vi "slider.vi"(0 "Slide":dbl(slide) scale=0.0..10.0, 6 "Playback":bool, 8 "Stop":bool, 11 "error in (no error)":errorcluster) -> (4 "Display Text":string caption="String 2", 15 "error out":errorcluster)   [LabVIEW 2023, in "Task_1.lvlib"]
doc: "Slider to set the value."
uses:
  Task_1.lvlib
  Control/Operations.ctl
  Control/Data.ctl
  Control/Control 7.ctl
  Control/State.ctl
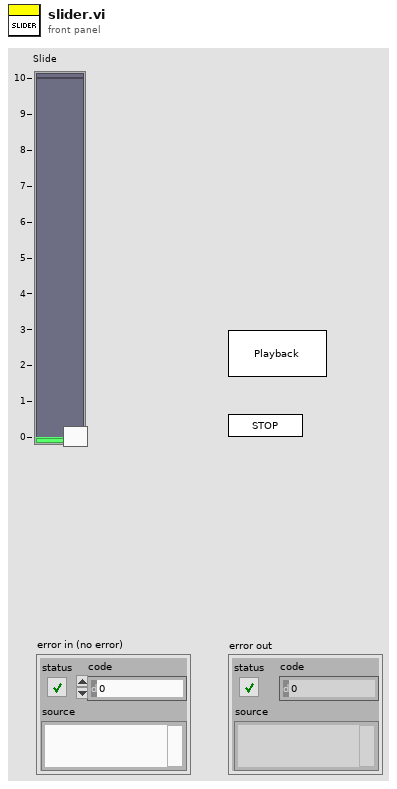
[diagram p1: front panel]
types:
  T1 = typedef "Control 7.ctl" = cluster{"State":T2, "Data":dbl[], "Index":i32}
  T2 = typedef "Task_1.lvlib/State.ctl" = enum16{"Idle", "Playback", "Record"}
  T3 = typedef "Task_1.lvlib/Data.ctl" = cluster{"Created?":bool, "Data":dbl}
  T4 = typedef "Task_1.lvlib/Operations.ctl" = enum16{"Create", "Gen_ref", "Generate", "Destroy"}
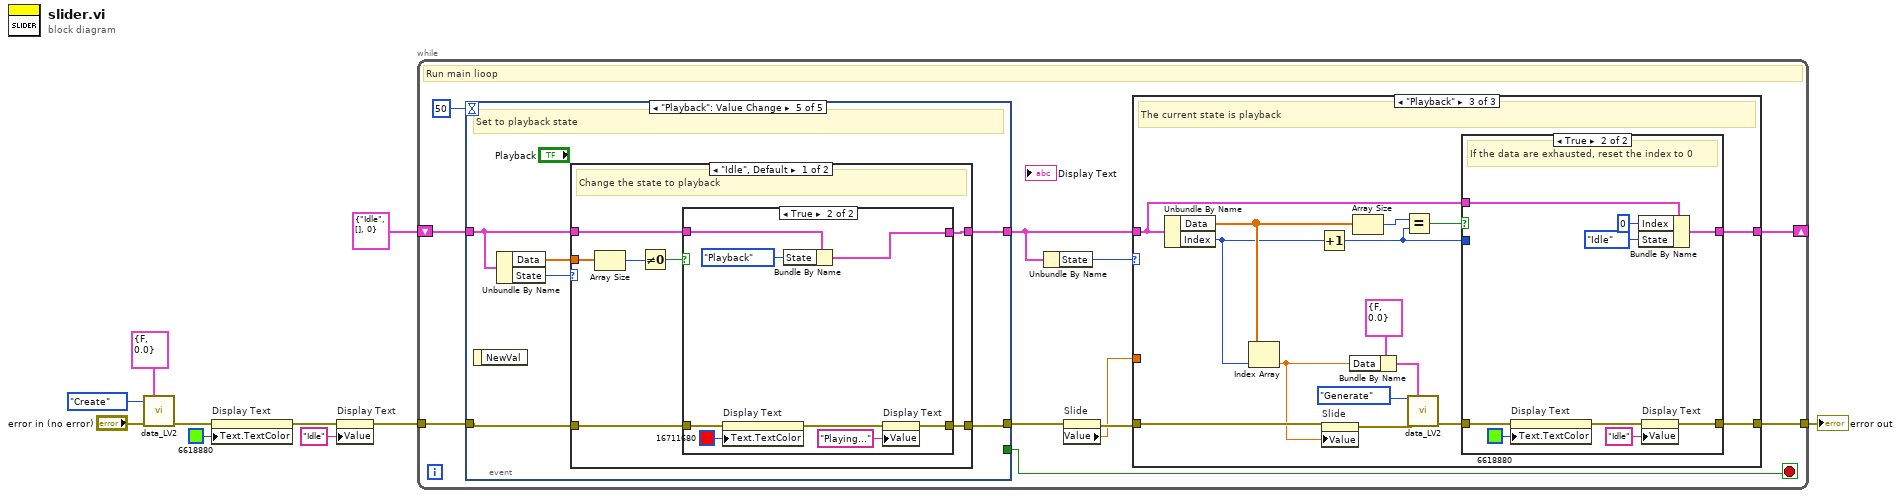
[diagram p0: block diagram]
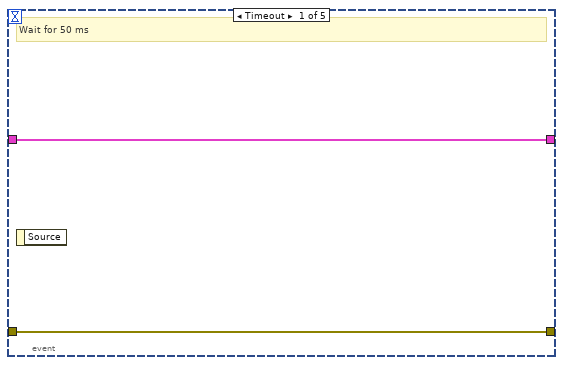
[diagram p2: hidden frame]
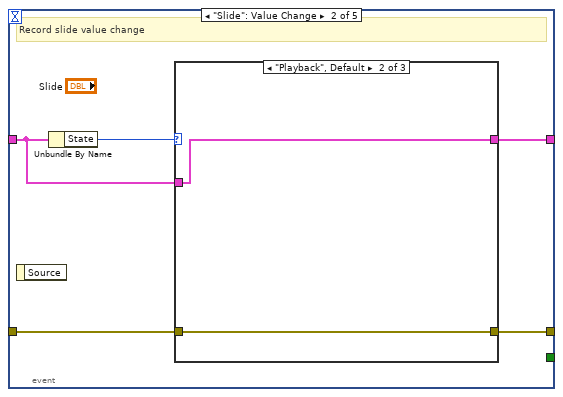
[diagram p3: hidden frame]
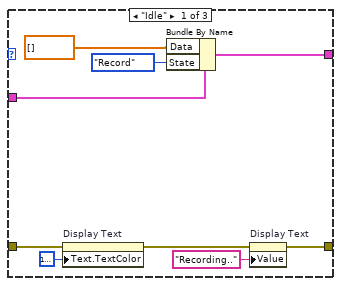
[diagram p4: hidden frame]
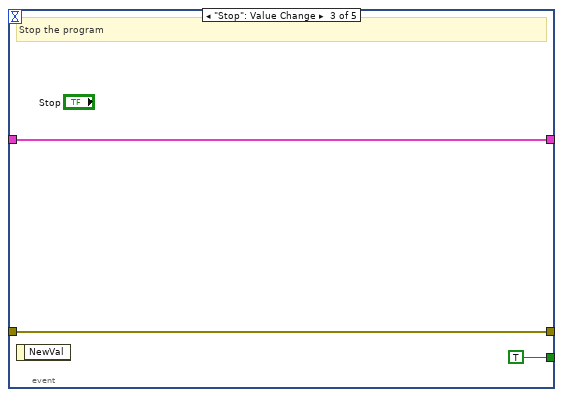
[diagram p6: hidden frame]
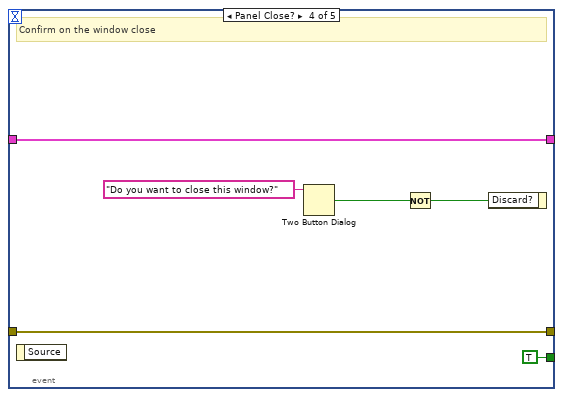
[diagram p7: hidden frame]
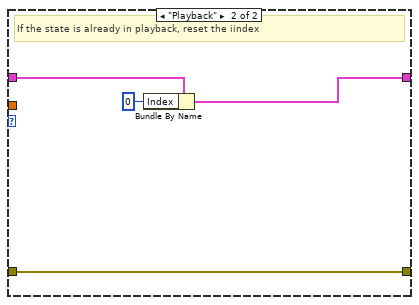
[diagram p9: hidden frame]
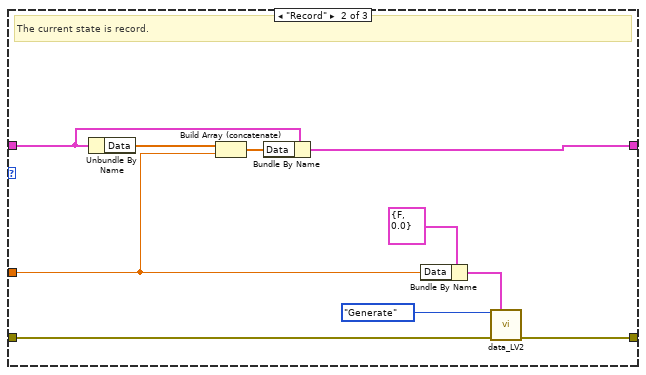
[diagram p11: hidden frame]
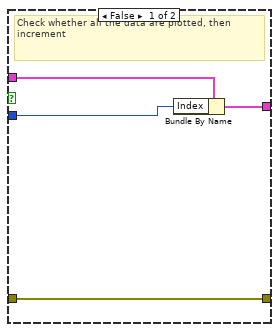
[diagram p12: hidden frame]
diagram:
  n1 = call "data_LV2.vi"("Option"=Operations."Create", "Data"=T3 {"Created?"=FALSE, "Data"=0.0}, "error in (no error)"="error in (no error)") -> ("error out"=w1:errorcluster)  [unwired: 11 in, 1 out]
  n2 = property on="Display Text" class="Str"(error in=w1, "Text.TextColor"=u32 6618880 ("Text.Text Colors:Text Color")) -> (error out=w4:errorcluster)  [unwired: 1 in, 1 out]
  n3 = property on="Display Text" class="Str"(error in=w4, "Value"="Idle" ("Display Text")) -> (error out=w2:errorcluster)  [unwired: 1 in, 1 out]
  n4 = while {
    tunnel: w2 -> [w13]
    tunnel: [w17] -> w9
    shift-right: [w16] -> _
    shift-left: T1 {"State"=enum."Idle", "Data"=[], "Index"=0} -> [w21]
    stop <- w11 stop-if-true
    # "Run main lioop"
    n5 = event shown="[4] \"Playback\": Value Change" {
      selector: _ -> [_ _ _ _ _]
      dyn-events: _ -> [_ _ _ _ _]
      timeout: 50 -> [_ _ _ _ _]
      tunnel: w21 -> [w23 w27 w44 w50 w55]
      tunnel: [w23 w26 w44 w50 w56] -> w15
      tunnel: w13 -> [w22 w25 w43 w49 w53]
      tunnel: [w22 w24 w43 w49 w52] -> w12
      tunnel: [_ _ TRUE TRUE _] -> w11
      event Timeout {
        # "Wait for 50 ms"
        n6 = event-data() -> ()  [unwired: 1 in, 1 out]
      }
      event "Slide": Value Change {
        # "Record slide value change"
        n7 = event-data() -> ()  [unwired: 1 in, 1 out]
        n8 = Unbundle By Name(w27) -> ("State"=w28:T2)
        n9 = case shown="\"Playback\", Default" w28 {
          tunnel: w27 -> [w37 w39 w41]
          tunnel: [w35 w39 w41] -> w26
          tunnel: w25 -> [w29 w38 w40]
          tunnel: [w30 w38 w40] -> w24
          frame "Idle" {
            n10 = property on="Display Text" class="Str"(error in=w29, "Text.TextColor"=u32 16777222 ("Text.Text Colors:Text Color")) -> (error out=w33:errorcluster)  [unwired: 1 in, 1 out]
            n11 = Bundle By Name(cluster=w37, "Data"=dbl[] [], "State"=State."Record") -> (w35:T1)
            n12 = property on="Display Text" class="Str"(error in=w33, "Value"="Recording.." ("Display Text")) -> (error out=w30:errorcluster)  [unwired: 1 in, 1 out]
          }
          frame "Playback", Default {
          }
          frame "Record" {
          }
        }
      }
      event "Stop": Value Change {
        # "Stop the program"
        n13 = event-data() -> ()  [unwired: 1 in, 1 out]
      }
      event Panel Close? {
        # "Confirm on the window close"
        n14 = event-data() -> ()  [unwired: 1 in, 1 out]
        n15 = Two Button Dialog(message="Do you want to close this window?") -> (T button?=w47:bool)  [unwired: 2 in]
        n16 = Not(x=w47) -> (.not. x?=w45:bool)
        n17 = event-data("Discard?"=w45) -> ()  [unwired: 1 in, 1 out]
      }
      event "Playback": Value Change {
        # "Set to playback state"
        n18 = event-data() -> ()  [unwired: 1 in, 1 out]
        n19 = Unbundle By Name(w55) -> ("Data"=w51:dbl[], "State"=w54:T2)
        n20 = case shown="\"Idle\", Default" w54 {
          tunnel: w55 -> [w60 w77]
          tunnel: [w63 w76] -> w56
          tunnel: w53 -> [w62 w74]
          tunnel: [w61 w74] -> w52
          tunnel: w51 -> [w59 _]
          frame "Idle", Default {
            # "Change the state to playback"
            n21 = Array Size(array=w59) -> (size(s)=w57:i32)
            n22 = Not Equal To 0?(x=w57) -> (x != 0?=w58:bool)
            n23 = case shown="True" w58 {
              tunnel: w60 -> [w65 w73]
              tunnel: [w65 w72] -> w63
              tunnel: w62 -> [w64 w67]
              tunnel: [w64 w66] -> w61
              frame False {
              }
              frame True {
                n24 = property on="Display Text" class="Str"(error in=w67, "Text.TextColor"=u32 16711680 ("Text.Text Colors:Text Color")) -> (error out=w69:errorcluster)  [unwired: 1 in, 1 out]
                n25 = Bundle By Name(cluster=w73, "State"=State."Playback") -> (w72:T1)
                n26 = property on="Display Text" class="Str"(error in=w69, "Value"="Playing..." ("Display Text")) -> (error out=w66:errorcluster)  [unwired: 1 in, 1 out]
              }
            }
          }
          frame "Playback" {
            # "If the state is already in playback, reset the iindex"
            n27 = Bundle By Name(cluster=w77, "Index"=0) -> (w76:T1)
          }
        }
      }
    }
    n28 = Unbundle By Name(w15) -> ("State"=w14:T2)
    n29 = property on="Slide" class="Slide (strict)"(error in=w12) -> (error out=w19:errorcluster, "Value"=w18:dbl)  [unwired: 1 in, 1 out]
    n30 = case shown="\"Playback\"" w14 {
      tunnel: w19 -> [w78 w86 w91]
      tunnel: [w78 w85 w97] -> w17
      tunnel: w18 -> [_ w80 _]
      tunnel: w15 -> [w79 w82 w100]
      tunnel: [w79 w83 w101] -> w16
      frame "Idle", Default {
        # "The current state is idle"
      }
      frame "Record" {
        # "The current state is record."
        n31 = Unbundle By Name(w82) -> ("Data"=w81:dbl[])
        n32 = Build Array (concatenate)(w81, w80) -> (w84:dbl[])
        n33 = Bundle By Name(cluster=w82, "Data"=w84) -> (w83:T1)
        n34 = Bundle By Name(cluster=T3 {"Created?"=FALSE, "Data"=0.0} ("Data"), "Data"=w80) -> (w88:T3)
        n35 = call "data_LV2.vi"("Option"=Operations."Generate", "Data"=w88, "error in (no error)"=w86) -> ("error out"=w85:errorcluster)  [unwired: 11 in, 1 out]
      }
      frame "Playback" {
        # "The current state is playback"
        n36 = Unbundle By Name(w100) -> ("Data"=w96:dbl[], "Index"=w95:i32)
        n37 = Index Array(array=w96, index=w95) -> (element=w90:dbl)
        n38 = Increment(x=w95) -> (x+1=w93:i32)
        n39 = property on="Slide" class="Slide (strict)"(error in=w91, "Value"=w90) -> (error out=w92:errorcluster)  [unwired: 1 in, 1 out]
        n40 = Bundle By Name(cluster=T3 {"Created?"=FALSE, "Data"=0.0} ("Data"), "Data"=w90) -> (w103:T3)
        n41 = Array Size(array=w96) -> (size(s)=w94:i32)
        n42 = Equal?(x=w94, y=w93) -> (x = y?=w99:bool)
        n43 = call "data_LV2.vi"("Option"=Operations."Generate", "Data"=w103, "error in (no error)"=w92) -> ("error out"=w98:errorcluster)  [unwired: 11 in, 1 out]
        n44 = case shown="True" w99 {
          tunnel: [w108 w116] -> w101
          tunnel: w100 -> [w107 w117]
          tunnel: w93 -> [w106 _]
          tunnel: w98 -> [w105 w112]
          tunnel: [w105 w111] -> w97
          frame False {
            # "Check whether all the data are plotted, then increment"
            n45 = Bundle By Name(cluster=w107, "Index"=w106) -> (w108:T1)
          }
          frame True {
            # "If the data are exhausted, reset the index to 0"
            n46 = property on="Display Text" class="Str"(error in=w112, "Text.TextColor"=u32 6618880 ("Text.Text Colors:Text Color")) -> (error out=w110:errorcluster)  [unwired: 1 in, 1 out]
            n47 = Bundle By Name(cluster=w117, "Index"=0, "State"=State."Idle") -> (w116:T1)
            n48 = property on="Display Text" class="Str"(error in=w110, "Value"="Idle" ("Display Text")) -> (error out=w111:errorcluster)  [unwired: 1 in, 1 out]
          }
        }
      }
    }
  }
  "error out" <- w9
